vi "add_scope_waveforms.vi"(8 "Error in (no error)":errorcluster, 11 "Waveform array":waveform(dbl)[](array[waveform])) -> (0 "Error out":errorcluster, 3 "Summed waveform":waveform(dbl))   [LabVIEW 2023]
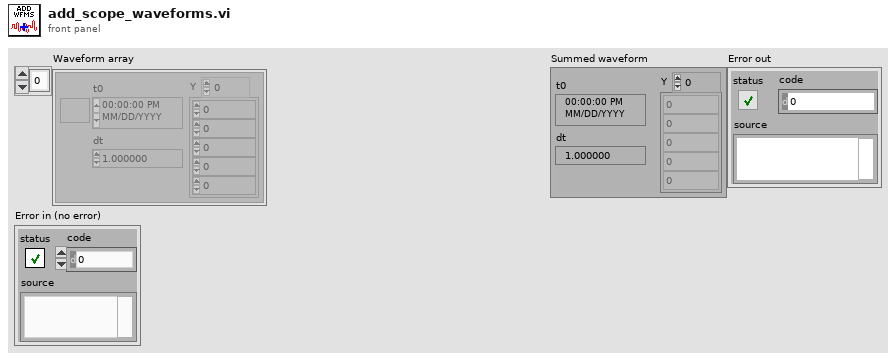
[diagram p1: front panel]
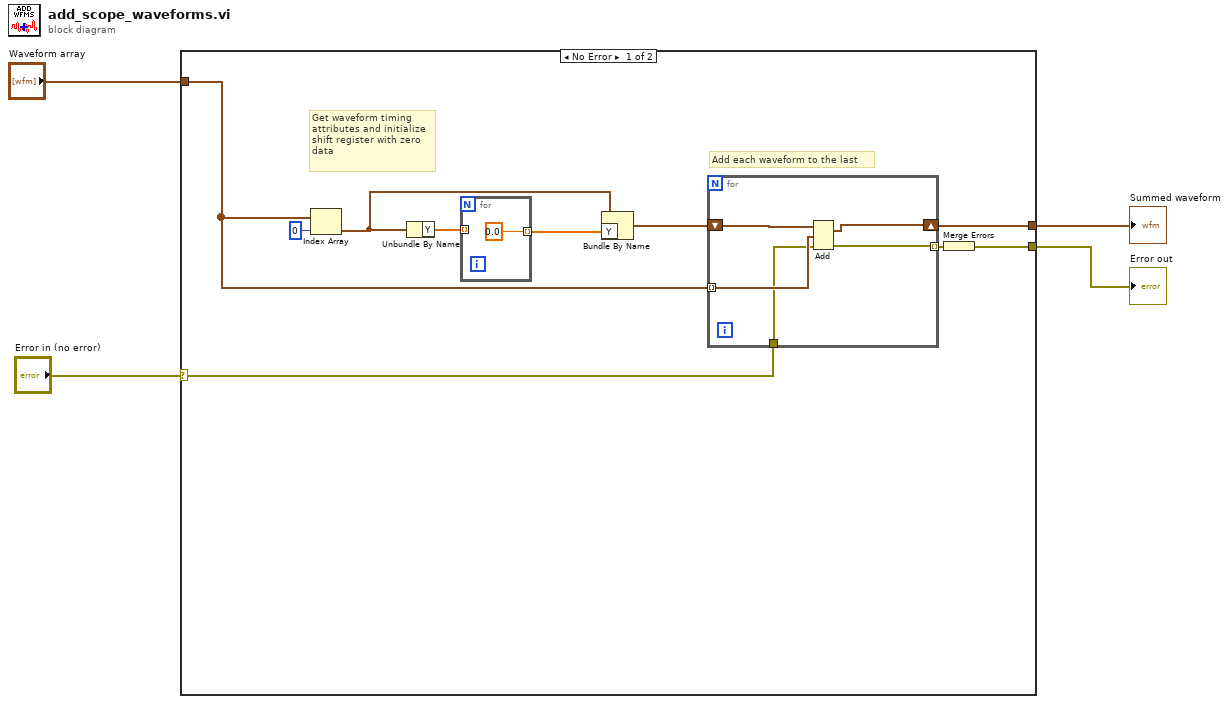
[diagram p0: block diagram]
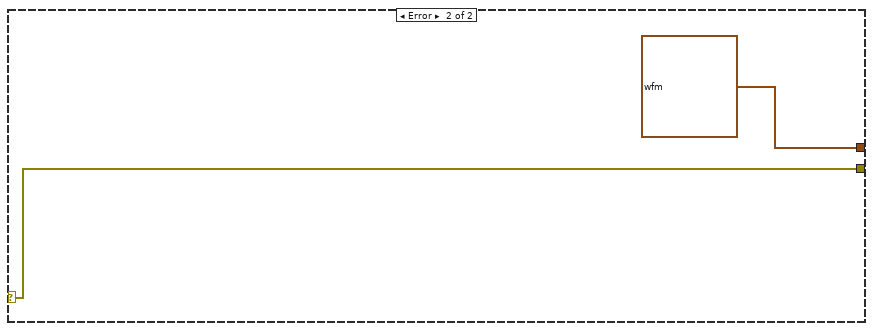
[diagram p2: hidden frame]
diagram:
  n1 = case shown="No Error" "Error in (no error)" {
    selector: "Error in (no error)" -> [w8 w22]
    tunnel: "Waveform array" -> [w9 _]
    tunnel: [w6 w22] -> w1
    tunnel: [w5 waveform(dbl) {"t0"=timestamp(0 s since 1904-01-01), "dt"=1.0, "Y"=[]} ("Waveform")] -> w2
    frame No Error {
      # "Add each waveform to the last"
      # "Get waveform timing \nattributes and initialize \nshift register with zero\ndata"
      n2 = Index Array(array=w9, index=0) -> (element=w11:waveform(dbl))
      n3 = Unbundle By Name(w11) -> ("Y"=w13:dbl[])
      n4 = for {
        tunnel: w13 -> [_] mode=indexing
        tunnel: [0.0] -> w12 mode=indexing
      }
      n5 = Bundle By Name(cluster=w11, "Y"=w12) -> (w10:waveform(dbl))
      n6 = for {
        shift-right: [w18] -> w5
        shift-left: w10 -> [w19]
        tunnel: w9 -> [w17] mode=indexing
        tunnel: w8 -> [w16]
        tunnel: [w15] -> w7 mode=indexing
        n7 = Add(1:w17, 2:w19, 4:w16) -> (0:w18:waveform(dbl), 3:w15:errorcluster)
      }
      n8 = Merge Errors(w7) -> (w6:errorcluster)
    }
    frame Error {
    }
  }
  "Summed waveform" <- w2
  "Error out" <- w1
